vi "Pop Up.vi"(10 "Pop Up":bool, 11 "Dev Panel in":refnum<class "Dev Panel.lvclass">) -> (0 "error out":errorcluster)   [LabVIEW 2021, in "Dev Panel.lvclass"]
uses:
  Dev Panel.lvclass
  Dev Panel.lvclass/Dev Panel.ctl
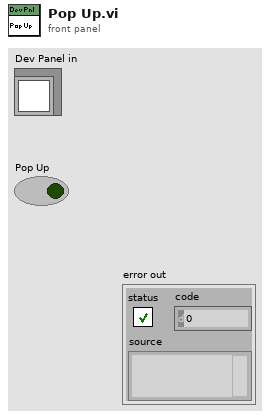
[diagram p1: front panel]
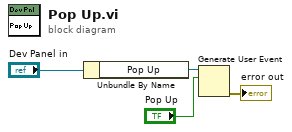
[diagram p0: block diagram]
diagram:
  n1 = Unbundle By Name("Dev Panel in") -> ("Pop Up"=w3:refnum<user-event>)
  n2 = Generate User Event(user event=w3, event data cluster="Pop Up") -> (error out=→"error out":errorcluster)  [unwired: 2 in, 1 out]
